vi "ziModGetData.vi"   [LabVIEW 2009, in "Zurich Instruments LabOne.lvlib"]
uses:
  <instrlib>/Zurich Instruments LabOne/Zurich Instruments LabOne.lvlib
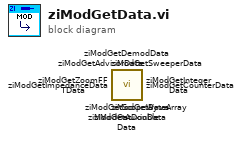
[diagram p0: block diagram]
diagram:
  n1 = call <instrlib>:"ziModGetScopeWave.vi"() -> ()  [unwired: 8 in, 4 out]
  n2 = call <instrlib>:"ziModGetSweeperData.vi"() -> ()  [unwired: 7 in, 5 out]
  n3 = call <instrlib>:"ziModGetImpedanceData.vi"() -> ()  [unwired: 8 in, 4 out]
  n4 = call <instrlib>:"ziModGetCounterData.vi"() -> ()  [unwired: 9 in, 3 out]
  n5 = call <instrlib>:"ziModGetAuxinData.vi"() -> ()  [unwired: 8 in, 4 out]
  n6 = call <instrlib>:"ziModGetDemodData.vi"() -> ()  [unwired: 8 in, 4 out]
  n7 = call <instrlib>:"ziModGetAdvisorData.vi"() -> ()  [unwired: 9 in, 3 out]
  n8 = call <instrlib>:"ziModGetByteArray.vi"() -> ()  [unwired: 9 in, 3 out]
  n9 = call <instrlib>:"ziModGetZoomFFTData.vi"() -> ()  [unwired: 9 in, 3 out]
  n10 = call <instrlib>:"ziModGetIntegerData.vi"() -> ()  [unwired: 7 in, 5 out]
  n11 = call <instrlib>:"ziModGetDoubleData.vi"() -> ()  [unwired: 7 in, 5 out]
